vi "鼠标离开标题读取.vi"(4 "error in (no error)":errorcluster, 6 "Container State":T2, 7 "Display State In":T1) -> (0 "error out":errorcluster, 2 "Value":string caption="鼠标读取离开标题", 3 "Display State Out":T1)   [LabVIEW 2011, in "ChangeColorBtn.xctl"]
uses:
  ChangeColorBtn.xctl
  <vilib>/_xctls/Container State.ctl
  State 1.ctl
  <vilib>/_xctls/XControlSupport.lvlib
panel:
  # "Replace the Value Indicator below with an Indicator of desired type.\nDo not remove this Indicator or the others from the connector pane. \nDo not change the connector pane pattern.\nThe Value Indicator should always be the second terminal from top on the output side in the connector pane."
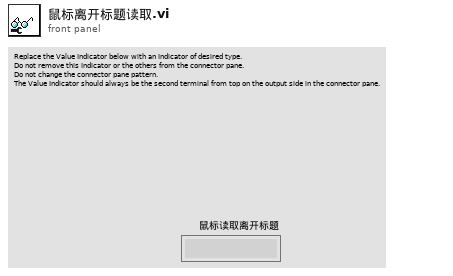
[diagram p1: front panel]
types:
  T1 = typedef "ChangeColorBtn.xctl/State 1.ctl" = cluster{"鼠标进入标题":string, "鼠标离开标题":string, "鼠标进入颜色":cluster{"Color Box":u32, "Color Box 2":u32}[], "鼠标离开颜色":cluster{"Color Box":u32, "Color Box 2":u32}[]}
  T2 = typedef "XControlSupport.lvlib/Container State.ctl" = cluster{"Indicator?":bool, "Run Mode?":bool, " Refnum":refnum<vi>}
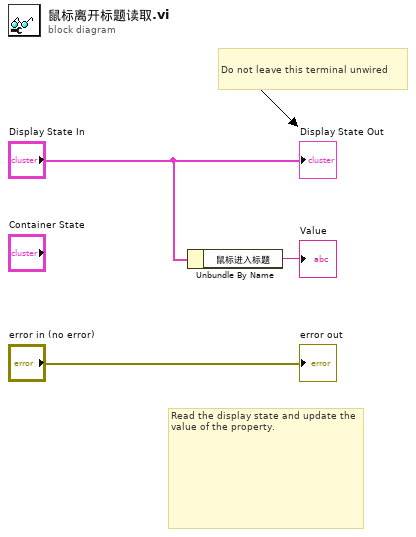
[diagram p0: block diagram]
diagram:
  # "Do not leave this terminal unwired"
  # "Read the display state and update the value of the property."
  n1 = Unbundle By Name("Display State In") -> ("鼠标进入标题"=→"Value":string)
  "error out" <- "error in (no error)"
  "Display State Out" <- "Display State In"
